vi "Post Exec Callout.vi"(8 "error in (no error)":errorcluster, 11 "RST in":refnum<class "RST.lvclass">) -> (0 "error out":errorcluster, 3 "RST out":refnum<class "RST.lvclass">)   [LabVIEW 2023, in "HAF.lvlib" / "RST.lvclass"]
doc: "Called at the end of the Processing of a specific Command so that additional code can be run. \n\nWhen the Reset command is run, any Driver Settings tht were applied to the Instrument are also reset. Need to reflect that back in the Driver Settings so that any follow-on Commands can commit them."
uses:
  RST.lvclass
  RST.lvclass/RST.ctl
  Driver/Driver.lvclass
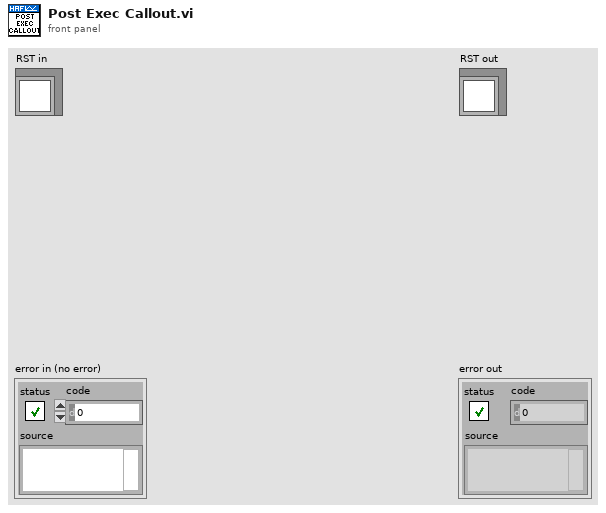
[diagram p1: front panel]
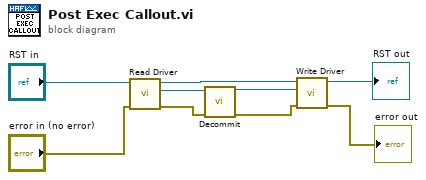
[diagram p0: block diagram]
diagram:
  n1 = call-dynamic "Read Driver.vi"("error in (no error)"="error in (no error)", "WriteCommand in"="RST in") -> ("error out"=w6:errorcluster, "Driver"=w7:refnum<class "Driver.lvclass">, "WriteCommand out"=w5:refnum<class "RST.lvclass">)  [unwired: 7 in]
  n2 = call-dynamic "Decommit.vi"("error in (no error)"=w6, "Driver in"=w7) -> ("error out"=w3:errorcluster, "Driver out"=w4:refnum<class "Driver.lvclass">)  [unwired: 8 in]
  n3 = call-dynamic "Write Driver.vi"("error in (no error)"=w3, "HAF:Driver.lvclass"=w4, "WriteCommand in"=w5) -> ("error out"=→"error out":errorcluster, "WriteCommand out"=→"RST out":refnum<class "RST.lvclass">)  [unwired: 7 in]
